vi "Copy Asset To Clipboard.vi"(8 "error in (no error)":errorcluster, 11 "Asset":T1) -> (0 "error out":errorcluster)   [LabVIEW 2019]
doc: "Attempt to copy the graphic specified by UID from BD Graphics.vi to the clipboard."
uses:
  Asset Enum.ctl
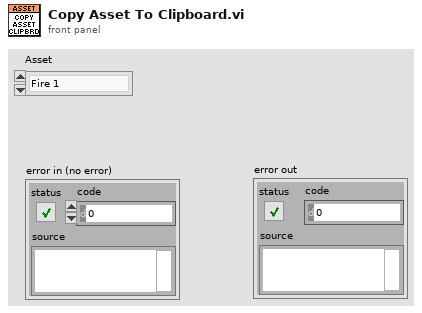
[diagram p1: front panel]
types:
  T1 = typedef "Asset Enum.ctl" = enum16{"Fire 1", "Fire 2", "Rubble"}
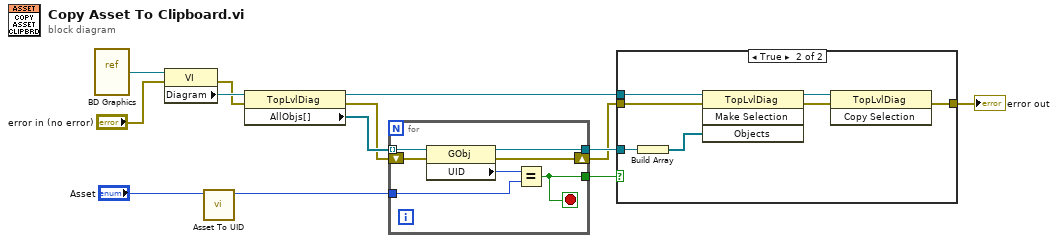
[diagram p0: block diagram]
diagram:
  n1 = vi-ref "BD Graphics.vi"() -> (w10:refnum<vi>)
  n2 = property class="VI"(reference=w10, error in="error in (no error)") -> (error out=w8:errorcluster, "Diagram"=w13:refnum<vi>)  [unwired: 1 out]
  n3 = call "Asset To UID.vi"("Asset"="Asset") -> ("UID"=w1:i32)  [unwired: 10 in]
  n4 = property class="TopLvlDiag"(reference=w13, error in=w8) -> (reference out=w11:refnum<vi>, error out=w7:errorcluster, "AllObjs[]"=w9:refnum<vi>[])
  n5 = for {
    tunnel: w9 -> [w20] mode=indexing
    tunnel: [w18] -> w12
    tunnel: w1 -> [w17]
    shift-right: [w15] -> w5
    shift-left: w7 -> [w16]
    tunnel: [w14] -> w6
    stop <- w14 stop-if-true
    n6 = property class="GObj"(reference=w20, error in=w16) -> (reference out=w18:refnum<vi>, error out=w15:errorcluster, "UID"=w19:i32)
    n7 = Equal?(x=w19, y=w17) -> (x = y?=w14:bool)
  }
  n8 = case shown="True" w6 {
    tunnel: w12 -> [_ w28]
    tunnel: w11 -> [_ w26]
    tunnel: w5 -> [w21 w23]
    tunnel: [w21 w22] -> w3
    frame False {
    }
    frame True {
      n9 = Build Array(w28) -> (w27:refnum<vi>[])
      n10 = invoke class="TopLvlDiag" method="Make Selection"(reference=w26, error in=w23, "Objects"=w27) -> (reference out=w25:refnum<vi>, error out=w24:errorcluster)  [unwired: 1 in, 2 out]
      n11 = invoke class="TopLvlDiag" method="Copy Selection"(reference=w25, error in=w24) -> (error out=w22:errorcluster)  [unwired: 1 in, 2 out]
    }
  }
  "error out" <- w3
